vi "Calculate Min Alt.vi"(7 "Meters?":bool, 10 "Buffer (0-1)":dbl, 11 "P (mb)":sgl) -> (2 "Max O2":dbl, 3 "Altitude":dbl)   [LabVIEW 2013]
doc: "Calculate a minimum alttitude using the West equation. The minimum altitude will be a function of the buffer, current oxygen content and the barometric pressure."
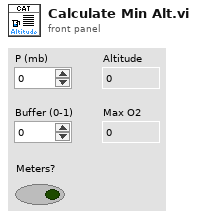
[diagram p1: front panel]
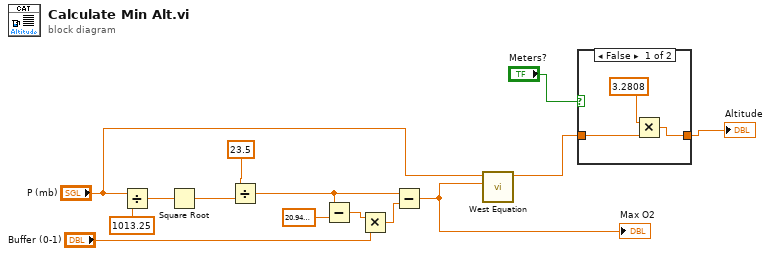
[diagram p0: block diagram]
diagram:
  n1 = Divide(x="P (mb)", y=sgl 1013.25) -> (x/y=w12:sgl)
  n2 = Square Root(x=w12) -> (sqrt(x)=w5:sgl)
  n3 = Divide(x=sgl 23.5, y=w5) -> (x/y=w10:sgl)
  n4 = Subtract(x=w10, y=sgl 20.94) -> (x-y=w9:sgl)
  n5 = Multiply(x=w9, y="Buffer (0-1)") -> (x*y=w8:dbl)
  n6 = Subtract(x=w10, y=w8) -> (x-y=w13:dbl)
  "Max O2" <- w13
  n7 = call "West Equation.vi"("O2%"=w13, "P (mb)"="P (mb)") -> ("Altitude (m)"=w2:dbl)  [unwired: 9 in]
  n8 = case shown="False" "Meters?" {
    tunnel: w2 -> [w17 w18]
    tunnel: [w15 w18] -> w1
    frame False {
      n9 = Multiply(x=3.2808, y=w17) -> (x*y=w15:dbl)
    }
    frame True {
    }
  }
  "Altitude" <- w1
